vi "SS2 Live_Init Recording.vi"(8 "Error In":errorcluster, 11 "SS2 Live Internal Variables in":T1={"okCFrontPanelDevices Refnum"=refnum, "Device Refnum"=refnum, "Display Image"=refnum, "# Live Images"=0, "relative s"=0.0, "# Image Sets"=0, "Message"="", "Current Image Set"=0, "# Datasets"=0, "Current Dataset"=0, "Live Mode"=FALSE, "Recording Mode"=FALSE, "Record Button"=refnum, "Live Button"=refnum, "SS2 Live Gate Data Q Name"="SS2 Live Gate Data Q", "Discard First Image"=FALSE, "Image Information"={"Save ROI Only"=FALSE, "Left"=0, "Top"=0, "Right"=0, "Bottom"=0, "Use Current ROI"=FALSE}, "Image Binning Options"={"Use Image Binning"=FALSE, "X Bin"=1, "Y Bin"=1}} {"Image Binning Options"."Y Bin" min=1; "Image Binning Options"."X Bin" min=1}) -> (0 "Error Out":errorcluster, 1 "Notebook Message":string, 3 "SS2 Live Internal Variables out":T1={"okCFrontPanelDevices Refnum"=refnum, "Device Refnum"=refnum, "Display Image"=refnum, "# Live Images"=0, "relative s"=0.0, "# Image Sets"=0, "Message"="", "Current Image Set"=0, "# Datasets"=0, "Current Dataset"=0, "Live Mode"=FALSE, "Recording Mode"=FALSE, "Record Button"=refnum, "Live Button"=refnum, "SS2 Live Gate Data Q Name"="SS2 Live Gate Data Q", "Discard First Image"=FALSE, "Image Information"={"Save ROI Only"=FALSE, "Left"=0, "Top"=0, "Right"=0, "Bottom"=0, "Use Current ROI"=FALSE}, "Image Binning Options"={"Use Image Binning"=FALSE, "X Bin"=1, "Y Bin"=1}} {"Image Binning Options"."Y Bin" min=1; "Image Binning Options"."X Bin" min=1})   [LabVIEW 2019]
uses:
  SS2 Live Internal Variables.ctl
  C:/UCLA Thinkpad Google Drive/LabVIEW 2019 SP1/builds/SS2 Live Distribution/Opal Kelly/C# Wrapper/libFrontPanel-csharp.dll
  Opal Kelly/C# Wrapper/libFrontPanel-csharp.dll
  <vilib>/vision/Image Controls.llb/IMAQ Image.ctl
  SS2 Live_Image ROI Information.ctl
  Phasor/Image Binning Options.ctl
  SS2 Live_Settings List.ctl
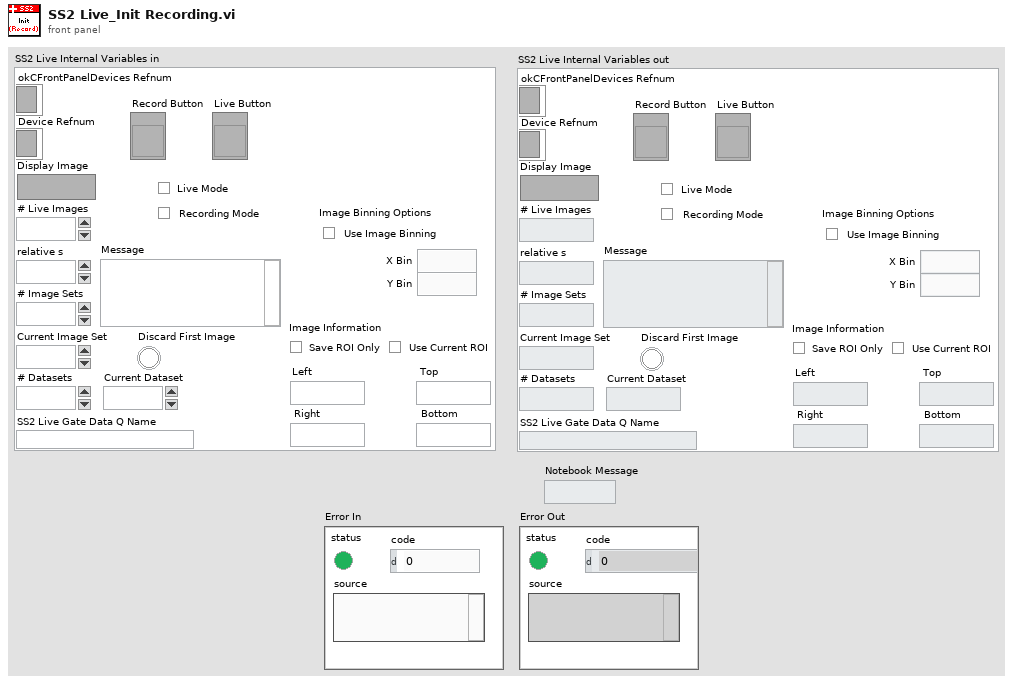
[diagram p1: front panel]
types:
  T1 = typedef "SS2 Live Internal Variables.ctl" = cluster{"okCFrontPanelDevices Refnum":refnum<k24>, "Device Refnum":refnum<k24>, "Display Image":T2, "# Live Images":i32, "relative s":dbl, "# Image Sets":i32, "Message":string, "Current Image Set":i32, "# Datasets":i32, "Current Dataset":i32, "Live Mode":bool, "Recording Mode":bool, "Record Button":refnum<vi>, "Live Button":refnum<vi>, "SS2 Live Gate Data Q Name":string, "Discard First Image":bool, "Image Information":T3, "Image Binning Options":T4}
  T2 = typedef "IMAQ Image.ctl" = refnum<image>
  T3 = typedef "SS2 Live_Image ROI Information.ctl" = cluster{"Save ROI Only":bool, "Left":u16, "Top":u16, "Right":u16, "Bottom":u16, "Use Current ROI":bool}
  T4 = typedef "Image Binning Options.ctl" = cluster{"Use Image Binning":bool, "X Bin":i32, "Y Bin":i32}
  T5 = typedef "SS2 Live_Settings List.ctl" = enum16{"FPGA:Bitfile Path", "FPGA:Bitfile Version", "Acquisition Parameters:SS2 DAQ Parameters", "Acquisition Parameters:Gate Configuration Array", "Acquisition Parameters:Buffer Size (# Gates)", "File Information:File Information", "File Information:# Datasets in Series", "Image Parameters:Image ROI Information", "Image Parameters:Image Binning Options", "UI Parameters:Histogram Bins Number"}
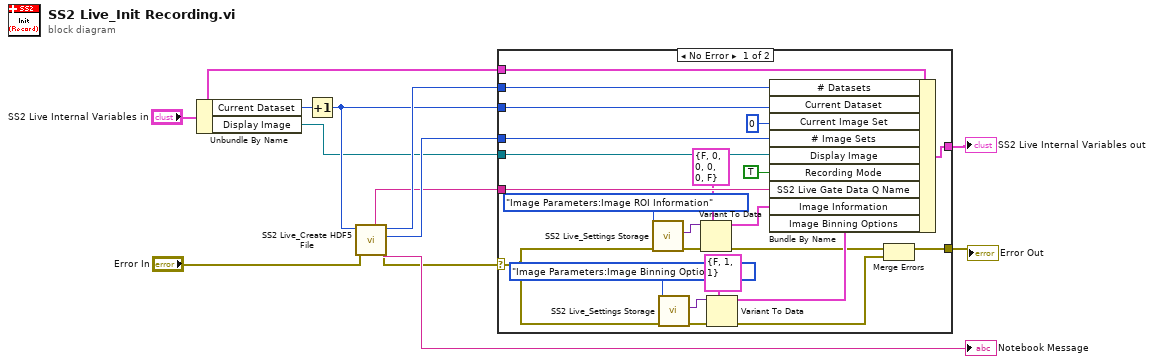
[diagram p0: block diagram]
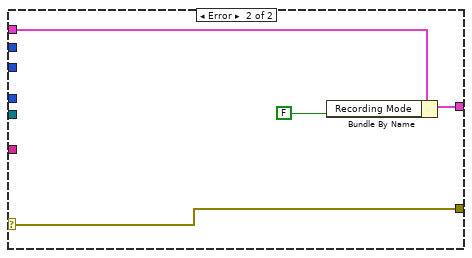
[diagram p2: hidden frame]
diagram:
  n1 = Unbundle By Name("SS2 Live Internal Variables in") -> ("Current Dataset"=w6:i32, "Display Image"=w1:T2)
  n2 = Increment(x=w6) -> (x+1=w5:i32)
  n3 = call "SS2 Live_Create HDF5 File.vi"("error in (no error)"="Error In", "Current Data Set"=w5) -> ("Error Out"=w2:errorcluster, "Notebook Message"=→"Notebook Message":string, "# Image Sets"=w8:u32, "# Data Sets"=w7:i32, "Data Q Name"=w4:string)  [unwired: 5 in]
  n4 = case shown="No Error" w2 {
    selector: w2 -> [w19 w36]
    tunnel: [w35 w38] -> w12
    tunnel: "SS2 Live Internal Variables in" -> [w34 w39]
    tunnel: w1 -> [w33 _]
    tunnel: w8 -> [w32 _]
    tunnel: w7 -> [w29 _]
    tunnel: w5 -> [w28 _]
    tunnel: w4 -> [w27 _]
    tunnel: [w14 w36] -> w3
    frame No Error {
      n5 = call "SS2 Live_Settings Storage.vi"("Error In"=w19, "Settings List"=SS2_Live_Settings_List."Image Parameters:Image ROI Information") -> ("Error Out"=w25:errorcluster, "Variant Data out"=w24:variant)  [unwired: 8 in]
      n6 = call "SS2 Live_Settings Storage.vi"("Error In"=w19, "Settings List"=SS2_Live_Settings_List."Image Parameters:Image Binning Options") -> ("Error Out"=w20:errorcluster, "Variant Data out"=w21:variant)  [unwired: 8 in]
      n7 = Variant To Data(error in=w25, type=T3 {"Save ROI Only"=FALSE, "Left"=0, "Top"=0, "Right"=0, "Bottom"=0, "Use Current ROI"=FALSE} ("Image Information"), Variant=w24) -> (data=w23:T3, error out=w15:errorcluster)
      n8 = Variant To Data(error in=w20, type=T4 {"Use Image Binning"=FALSE, "X Bin"=1, "Y Bin"=1} ("Image Binning Options"), Variant=w21) -> (data=w17:T4, error out=w13:errorcluster)
      n9 = Bundle By Name(cluster=w34, "# Datasets"=w29, "Current Dataset"=w28, "Current Image Set"=0, "# Image Sets"=w32, "Display Image"=w33, "Recording Mode"=TRUE, "SS2 Live Gate Data Q Name"=w27, "Image Information"=w23, "Image Binning Options"=w17) -> (w35:T1)
      n10 = Merge Errors(w15, w13) -> (w14:errorcluster)
    }
    frame Error {
      n11 = Bundle By Name(cluster=w39, "Recording Mode"=FALSE) -> (w38:T1)
    }
  }
  "SS2 Live Internal Variables out" <- w12
  "Error Out" <- w3
